vi "DCC_GetDLLPath.vi"(8 "Error In":errorcluster) -> (0 "Error Out":errorcluster, 3 "DLL Path":path, 4 "DCC Folder Path":path=path "C:/Program Files (x86)/BH/SPCM/DLL", 6 "Bit System":T1)   [LabVIEW 2019]
doc: "The \"DCC Get DLL Path Function\" checks whether the used system is a 32-bit or a 64-bit system and chooses the correct DLL path.\nNotice, that this function will use the default installation path. \nNormally, this is \"C:\\Program Files (x86)\\BH\\SPCM\\DLL\\\".\n\nOctober 2018\nFrank Quadt\ninfo@becker-hickl.com"
uses:
  <vilib>/registry/registry.llb/Registry View.ctl
  <vilib>/registry/registry.llb/Registry RtKey.ctl
  <vilib>/registry/registry.llb/Registry SAM.ctl
  <vilib>/registry/registry.llb/Read Registry Value Simple STR.vi
panel:
  out "32/64 subset":string="Substring containing \"32\" or \"64\""
  # "(c) 2021 Becker & Hickl GmbH\n     All Rights Reserved."
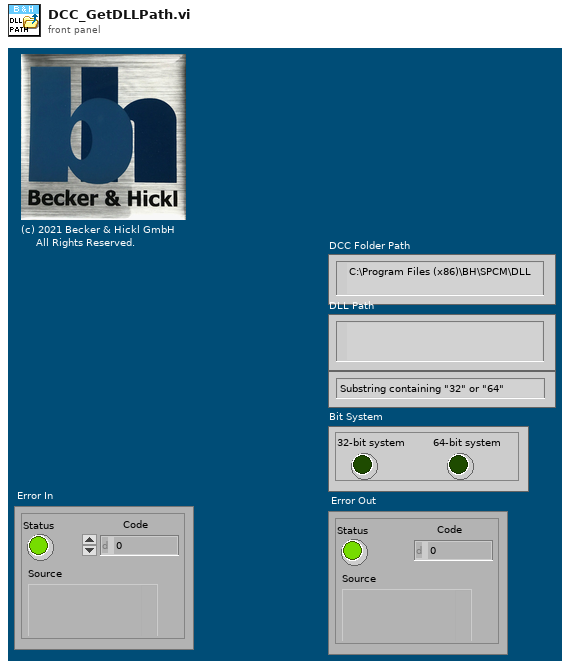
[diagram p1: front panel]
types:
  T1 = cluster{"32-bit system":bool, "64-bit system":bool}
  T2 = typedef "Registry SAM.ctl" = enum32{"KEY_QUERY_VALUE", "KEY_SET_VALUE", "KEY_CREATE_SUB_KEY", "KEY_ENUMERATE_SUB_KEYS", "KEY_NOTIFY", "KEY_CREATE_LINK", "KEY_READ", "KEY_WRITE", "KEY_ALL_ACCESS", "KEY_READ | KEY_WRITE"}
  T3 = typedef "Registry RtKey.ctl" = enum32{"HKEY_CLASSES_ROOT", "HKEY_CURRENT_USER", "HKEY_LOCAL_MACHINE", "HKEY_USERS", "HKEY_PERFORMANCE_DATA", "HKEY_CURRENT_CONFIG", "HKEY_DYN_DATA"}
  T4 = typedef "Registry View.ctl" = u16
  T5 = typedef "Registry refnum.ctl" = refnum<k1>
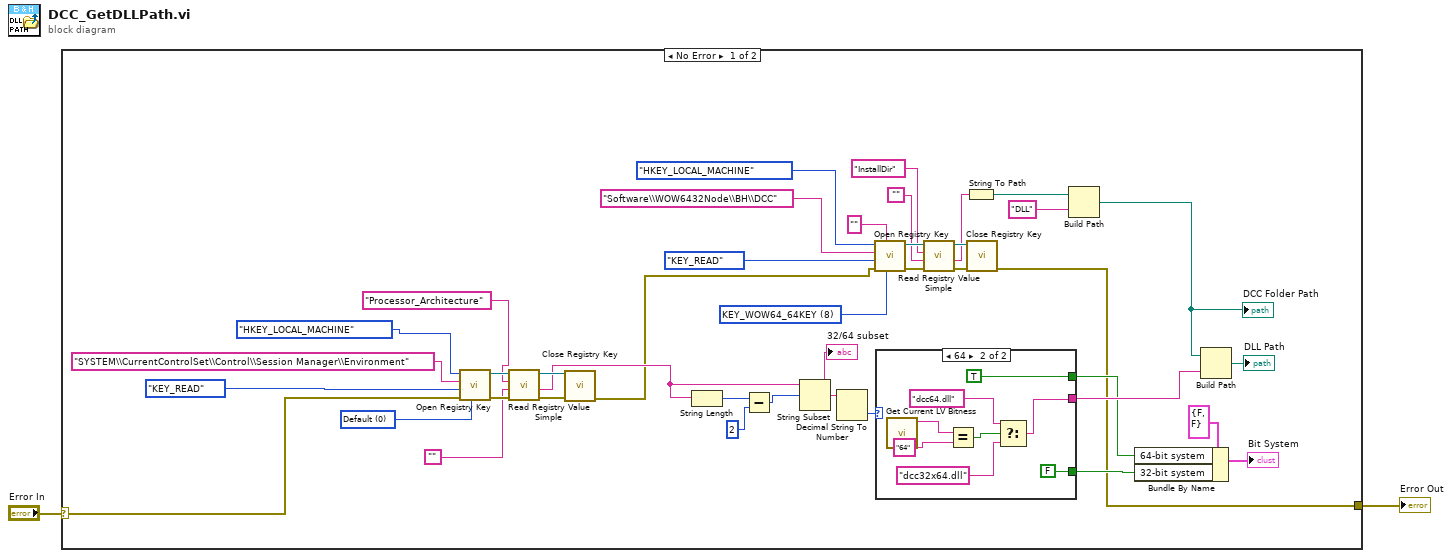
[diagram p0: block diagram]
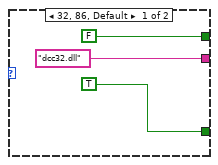
[diagram p2: hidden frame]
diagram:
  n1 = case shown="No Error" "Error In" {
    selector: "Error In" -> [w6 w54]
    tunnel: [w3 w54] -> w1
    frame No Error {
      w10 = T4 0 items=["Default"=0, "KEY_WOW64_64KEY"=8, "KEY_WOW64_32KEY"=9] ("registry view")
      w22 = T4 8 items=["Default"=0, "KEY_WOW64_64KEY"=8, "KEY_WOW64_32KEY"=9] ("registry view")
      n2 = call <vilib>:"Open Registry Key.vi"("registry view"=w10, "error in (no error)"=w6, "security access mask (KEY_READ | KEY_WRITE)"=Registry_SAM."KEY_READ", "subkey"="SYSTEM\\CurrentControlSet\\Control\\Session Manager\\Environment", "root key (HKEY_LOCAL_MACHINE)"=Registry_RtKey."HKEY_LOCAL_MACHINE") -> ("error out"=w16:errorcluster, "refnum out"=w15:T5)  [unwired: 5 in]
      n3 = call-poly <vilib>:"Read Registry Value Simple.vi"("error in (no error)"=w16, "default data"="", "value"="Processor_Architecture", "refnum"=w15) -> ("error out"=w14:errorcluster, "String/Binary data"=w5:string, "refnum out"=w13:T5)  [unwired: 2 in, 1 out]
      n4 = call <vilib>:"Close Registry Key.vi"("error in (no error)"=w14, "refnum"=w13) -> ("error out"=w4:errorcluster)  [unwired: 5 in]
      n5 = String Length(string=w5) -> (length=w42:i32)
      n6 = Subtract(x=w42, y=2) -> (x-y=w40:i32)
      n7 = String Subset(string=w5, offset (0)=w40) -> (substring=w38:string)  [unwired: 1 in]
      "32/64 subset" <- w38
      n8 = Decimal String To Number(string=w38) -> (number=w39:i32)  [unwired: 2 in, 1 out]
      n9 = call <vilib>:"Open Registry Key.vi"("registry view"=w22, "machine (local)"="", "error in (no error)"=w4, "security access mask (KEY_READ | KEY_WRITE)"=Registry_SAM."KEY_READ", "subkey"="Software\\WOW6432Node\\BH\\DCC", "root key (HKEY_LOCAL_MACHINE)"=Registry_RtKey."HKEY_LOCAL_MACHINE") -> ("error out"=w30:errorcluster, "refnum out"=w31:T5)  [unwired: 4 in]
      n10 = case shown="64" w39 {
        tunnel: [FALSE TRUE] -> w33
        tunnel: [TRUE FALSE] -> w34
        tunnel: ["dcc32.dll" w47] -> w37
        frame 32, 86, Default {
        }
        frame 64 {
          n11 = call <vilib>:"Get Current LV Bitness.vi"() -> ("bitness"=w46:string)  [unwired: 11 in]
          n12 = Equal?(x=w46, y="64") -> (x = y?=w51:bool)
          n13 = Select(t="dcc64.dll", s=w51, f="dcc32x64.dll") -> (s? t:f=w47:string)
        }
      }
      n14 = call-poly <vilib>:"Read Registry Value Simple.vi"("error in (no error)"=w30, "default data"="", "value"="InstallDir", "refnum"=w31) -> ("error out"=w28:errorcluster, "String/Binary data"=w26:string, "refnum out"=w29:T5)  [unwired: 2 in, 1 out]
      n15 = String To Path(string=w26) -> (path=w27:path)
      n16 = call <vilib>:"Close Registry Key.vi"("error in (no error)"=w28, "refnum"=w29) -> ("error out"=w3:errorcluster)  [unwired: 5 in]
      n17 = Build Path(base path=w27, name or relative path="DLL") -> (appended path=w17:path)
      "DCC Folder Path" <- w17
      n18 = Bundle By Name(cluster=T1 {"32-bit system"=FALSE, "64-bit system"=FALSE} ("Bit System 2"), "64-bit system"=w33, "32-bit system"=w34) -> (→"Bit System":T1)
      n19 = Build Path(base path=w17, name or relative path=w37) -> (appended path=→"DLL Path":path)
    }
    frame Error {
    }
  }
  "Error Out" <- w1
